vi "BasicFlow.vi"(0 "VI Reference In":refnum<vi>, 1 "Label (VI Title)":string="Default", 11 "error in (no error)":errorcluster) -> (4 "VI Reference Out":refnum<vi>, 15 "error out":errorcluster)   [LabVIEW 2016, in "DronaTest.lvlib"]
uses:
  DronaTest.lvlib
  main/apis/Stimulus/ValueSignal/ValueSignalByPathString.vi
  main/apis/Assert/AssertControlValue/Equal.vi
  <vilib>/addons/_JKI Toolkits/Caraya/classes/Assert/Assert Not Error.vi
  <vilib>/addons/_JKI Toolkits/Caraya/classes/Test/Test.lvclass
  main/Drona.lvlib
  <vilib>/addons/_JKI Toolkits/Caraya/classes/Assert/Assert.lvclass
  main/apis/Assert/AssertControlValue/AssertControlValue.lvlib
  main/apis/Stimulus/ValueSignal/ValueSignal.lvlib
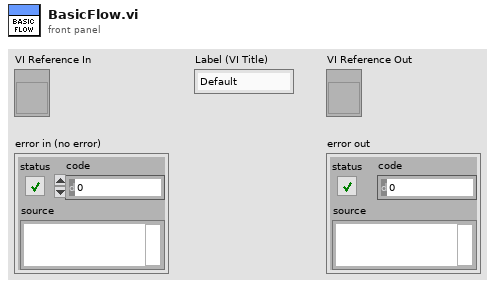
[diagram p1: front panel]
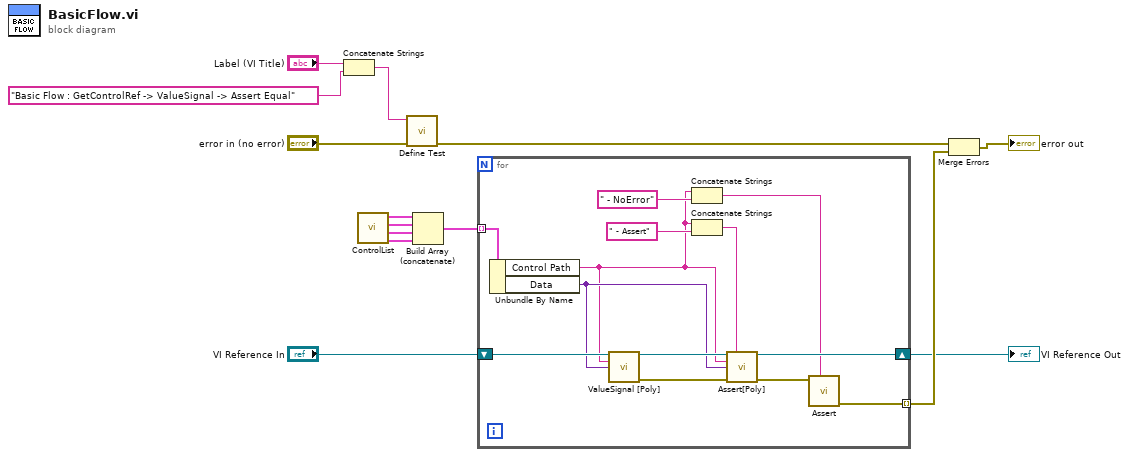
[diagram p0: block diagram]
diagram:
  n1 = Concatenate Strings("Label (VI Title)", "Basic Flow : GetControlRef -> ValueSignal -> Assert Equal" ("Label (VI Title)")) -> (w5:string)
  n2 = call "ControlList.vi"() -> ("Tab Control"=w1:cluster{"Control Path":string, "Data":variant}[], "BigCluster"=w2:cluster{"Control Path":string, "Data":variant}[], "Cluster"=w3:cluster{"Control Path":string, "Data":variant}[], "Basic"=w9:cluster{"Control Path":string, "Data":variant}[])  [unwired: 7 in, 1 out]
  n3 = call <vilib>:"Define Test.vi"("error in (no error)"="error in (no error)", "Label (VI Title)"=w5) -> ("error out"=w8:errorcluster)  [unwired: 9 in]
  n4 = Build Array (concatenate)(w9, w3, w2, w1) -> (w4:cluster{"Control Path":string, "Data":variant}[])
  n5 = for {
    shift-right: [w27] -> w11
    shift-left: "VI Reference In" -> [w23]
    tunnel: [w15] -> w14 mode=indexing
    tunnel: w4 -> [w24] mode=indexing
    n6 = Unbundle By Name(w24) -> ("Control Path"=w18:string, "Data"=w22:variant)
    n7 = call-poly "ValueSignal [Poly].vi"("VI Reference In"=w23, "Control Path"=w18, "Value (Signaling)"=w22) -> ("VI Reference Out"=w25:refnum<vi>, "error out"=w26:errorcluster)  [unwired: 11 in]
    n8 = Concatenate Strings(w18, " - NoError" ("string")) -> (w16:string)
    n9 = Concatenate Strings(w18, " - Assert" ("string")) -> (w20:string)
    n10 = call-poly "Assert[Poly].vi"("VI Reference In"=w25, "Label"=w20, "Control Path"=w18, "Control Value"=w22, "Error In"=w26) -> ("VI Reference Out"=w27:refnum<vi>, "Error Out"=w17:errorcluster)  [unwired: 9 in]
    n11 = call-poly <vilib>:"Assert.vi"("Label"=w16, "Not Error?"=w17) -> ("error out"=w15:errorcluster)  [unwired: 9 in]
  }
  "VI Reference Out" <- w11
  n12 = Merge Errors(w8, w14) -> (→"error out":errorcluster)
